vi "Build Model Data Cluster.vi"(1 "Model in":T1) -> (0 "Model out":T4)   [LabVIEW 2020, in "feature_detection.lvlib" / "Text Detector.lvclass"]
uses:
  Text Detector.lvclass
  Text Detector.lvclass/Text Detector.ctl
  common/Object Point (Float).ctl
  common/common.lvlib
  common/Image Size (Integer).ctl
  Model.ctl
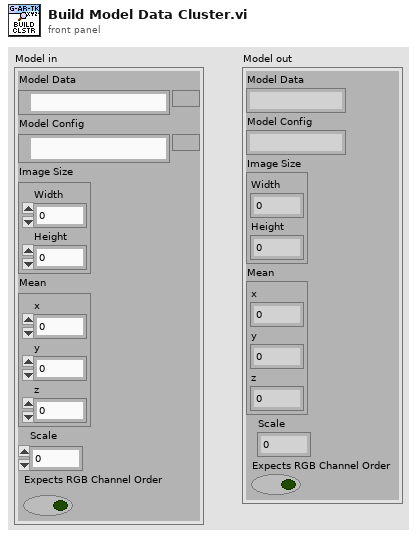
[diagram p1: front panel]
types:
  T1 = typedef "feature_detection.lvlib/Text Detector.lvclass/Model.ctl" = cluster{"Model Data":path, "Model Config":path, "Image Size":T2, "Mean":T3, "Scale":dbl, "Expects RGB Channel Order":bool}
  T2 = typedef "common.lvlib/Image Size (Integer).ctl" = cluster{"Width":u16, "Height":u16}
  T3 = typedef "common.lvlib/Object Point (Float).ctl" = cluster{"x":dbl, "y":dbl, "z":dbl}
  T4 = cluster{"Model Data":string, "Model Config":string, "Image Size":T2, "Mean":T3, "Scale":dbl, "Expects RGB Channel Order":bool}
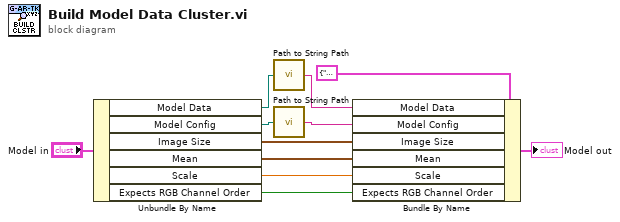
[diagram p0: block diagram]
diagram:
  n1 = Unbundle By Name("Model in") -> ("Model Data"=w5:path, "Model Config"=w3:path, "Image Size"=w6:T2, "Mean"=w7:T3, "Scale"=w8:dbl, "Expects RGB Channel Order"=w9:bool)
  n2 = call "Path to String Path.vi"("Path"=w5) -> ("String"=w4:string)
  n3 = call "Path to String Path.vi"("Path"=w3) -> ("String"=w2:string)
  n4 = Bundle By Name(cluster=T4 {"Model Data"="", "Model Config"="", "Image Size"={"Width"=0, "Height"=0}, "Mean"={"x"=0.0, "y"=0.0, "z"=0.0}, "Scale"=0.0, "Expects RGB Channel Order"=FALSE} ("Model"), "Model Data"=w4, "Model Config"=w2, "Image Size"=w6, "Mean"=w7, "Scale"=w8, "Expects RGB Channel Order"=w9) -> (→"Model out":T4)
